vi "Teleop.vi"(10 "Match Info":T1={"Autonomous Elapsed Seconds"=0.0, "TeleOp Elapsed Seconds"=0.0, "Disabled Elapsed Seconds"=0.0, "Visited Autonomous"=FALSE, "Visited TeleOp"=FALSE, "Visited Disabled"=FALSE, "Autonomous Settings"={"Autonomous Style"=enum."Independent", "VI Refnum"=refnum}}, 11 "Call Context":T2) -> ()   [LabVIEW 2017]
doc: "This VI is called for each TeleOp packet received from the DS where the robot is not disabled. It is often used to read from the joysticks and update I/O or to update setpoints for timed control loops. It should complete and return within 20 milliseconds or it may miss DS packets."
uses:
  <vilib>/Rock Robotics/WPI/DriverStation/WPI_DriverStationDerivedRobotMode.ctl
  <vilib>/Rock Robotics/WPI/DriverStation/WPI_DriverStationMatch Info.ctl
  Public/Documents/Cross The Road Electronics/Phoenix-LabVIEW/Pigeon IMU/CTRE_PigeonIMU_PigeonState.ctl
  <vilib>/Rock Robotics/WPI/Utilities/WPI_GetSetVariantRefNum.vi
  Public/Documents/Cross The Road Electronics/Phoenix-LabVIEW/Pigeon IMU/CTRE_PigeonIMU_GetFusedHeading.vi
  Public/Documents/Cross The Road Electronics/Phoenix-LabVIEW/Pigeon IMU/CTRE_PigeonIMU_GetTempStateUpTime.vi
  Public/Documents/Cross The Road Electronics/Phoenix-LabVIEW/Pigeon IMU/CTRE_PigeonIMU_GetRawGyro.vi
  <vilib>/Rock Robotics/Network Tables/NT Write Numeric Array.vi
panel:
  in  "D Gain":dbl=0.0004 format="%#_13g"
  in  "P Gain":dbl=0.04 format="%#_13g"
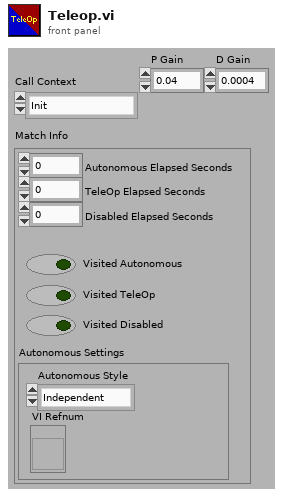
[diagram p1: front panel]
types:
  T1 = typedef "WPI_DriverStationMatch Info.ctl" = cluster{"Autonomous Elapsed Seconds":dbl, "TeleOp Elapsed Seconds":dbl, "Disabled Elapsed Seconds":dbl, "Visited Autonomous":bool, "Visited TeleOp":bool, "Visited Disabled":bool, "Autonomous Settings":cluster{"Autonomous Style":enum16{"Iterative", "Independent"}, "VI Refnum":refnum<vi>}}
  T2 = typedef "WPI_DriverStationDerivedRobotMode.ctl" = enum16{"Init", "Execute", "Stop"}
  T3 = typedef "WPI_RobotDriveDevRef.ctl" = cluster{"DevStatus":errorcluster, "Motors[]":T4[], "Square Inputs":bool, "Max Output":dbl}
  T4 = typedef "WPI_MotorControlDeviceRef.ctl" = cluster{"DeviceStatus":errorcluster, "Type":T5, "PWM":cluster{"PWM Channel":T6, "DeadBand":T7}, "CAN":cluster{"Device Number":u8, "SetOutput VI Ref":variant, "GetOutput VI Ref":variant, "Enable VI Ref":variant, "Disable VI Ref":variant, "Data":variant}, "Invert":bool, "DIO PWM":cluster{"PWM \"Enable\" Channel":T6, "DIOChannel":T8, "PWM Rate":dbl}}
  T5 = typedef "WPI_MotorControlType.ctl" = enum16{"PWM", "CAN", "DIO PWM"}
  T6 = typedef "FPGA_DIOPWMChannel.ctl" = enum8{"PWM 0", "PWM 1", "PWM 2", "PWM 3", "PWM 4", "PWM 5", "PWM 6", "PWM 7", "PWM 8", "PWM 9", "PWM MXP 0", "PWM MXP 1", "PWM MXP 2", "PWM MXP 3", "PWM MXP 4", "PWM MXP 5", "PWM MXP 6", "PWM MXP 7", "PWM MXP 8", "PWM MXP 9", "Invalid"}
  T7 = typedef "WPI_PWMDeadband.ctl" = cluster{"Name":string, "maxPositivePwm":i32, "minPositivePwm":i32, "centerPwm":i32, "maxNegativePwm":i32, "minNegativePwm":i32, "angularRange":u16}
  T8 = typedef "FPGA_DIOChannel.ctl" = enum8{"DIO 0", "DIO 1", "DIO 2", "DIO 3", "DIO 4", "DIO 5", "DIO 6", "DIO 7", "DIO 8", "DIO 9", "DIO MXP 0", "DIO MXP 1", "DIO MXP 2", "DIO MXP 3", "DIO MXP 4", "DIO MXP 5", "DIO MXP 6", "DIO MXP 7", "DIO MXP 8", "DIO MXP 9", "DIO MXP 10", "DIO MXP 11", "DIO MXP 12", "DIO MXP 13", "DIO MXP 14", "DIO MXP 15", "SPI Port CS1", "SPI Port CS2", "SPI Port CS3", "SPI Port MISO", "SPI Port MOSI", "Invalid"}
  T9 = typedef "WPI_JoystickDevRef.ctl" = cluster{"Device":T10}
  T10 = typedef "WPI_JoystickDeviceEnum.ctl" = enum16{"USB 0", "USB 1", "USB 2", "USB 3", "USB 4", "USB 5"}
  T11 = typedef "CTRE_PigeonIMU_DeviceRef.ctl" = cluster{"DeviceStatus":errorcluster, "Device Number":u8, "Type":T12, "Device ID":u32, "Handle":u64, "UsageFrame":u32, "Library Path":path}
  T12 = typedef "CTRE_PigeonIMU_ConnectionType.ctl" = u32
  T13 = typedef "CTRE_PigeonIMU_PigeonState.ctl" = enum16{"NoComm", "Initializing", "Ready", "UserCalibration"}
  T14 = cluster{"Heading":dbl, "Valid?":bool, "Fusing?":bool}
  T15 = typedef "CTRE_PigeonIMU_CalibrationMode.ctl" = u16
  T16 = cluster{"CurrentMode":T15, "LastCalError":i32, "CalBooting?":bool, "PigeonState":T13, "UpTime":u32, "Temp. (C)":dbl, "Temp Compensation Event Count":u32, "No Motion Event Count":u32}
  T17 = cluster{"X":dbl, "Y":dbl, "Z":dbl, "Magnitude":dbl}
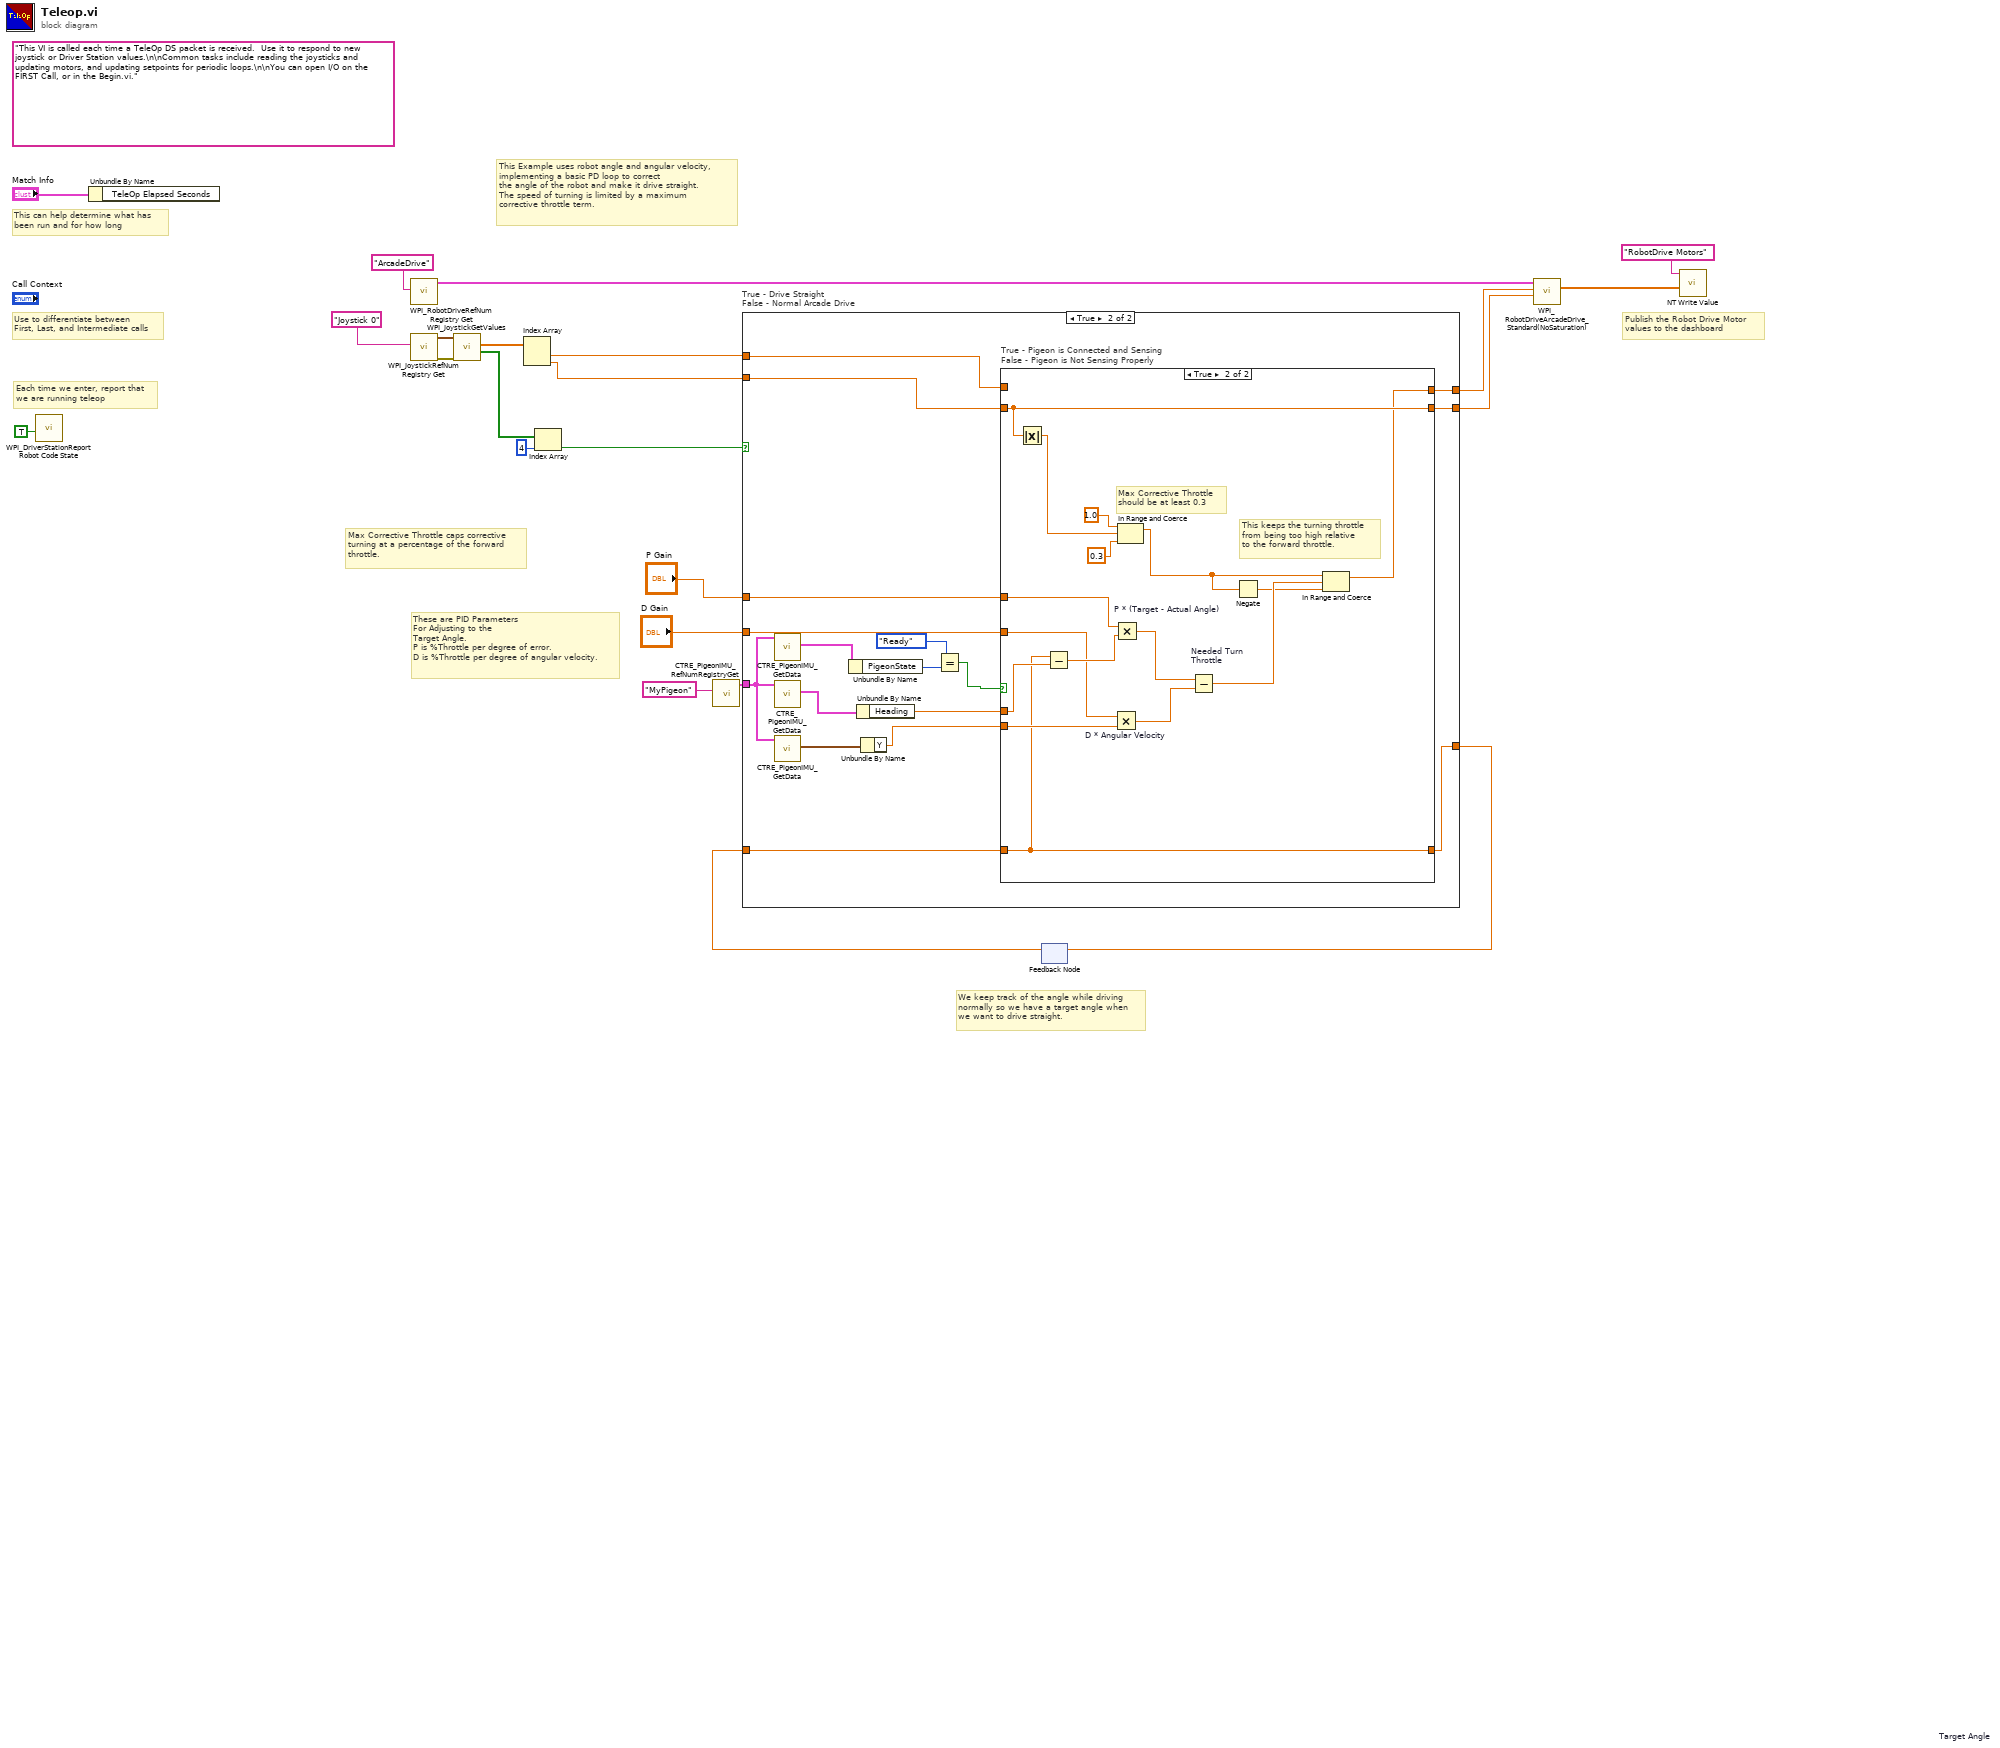
[diagram p0: block diagram]
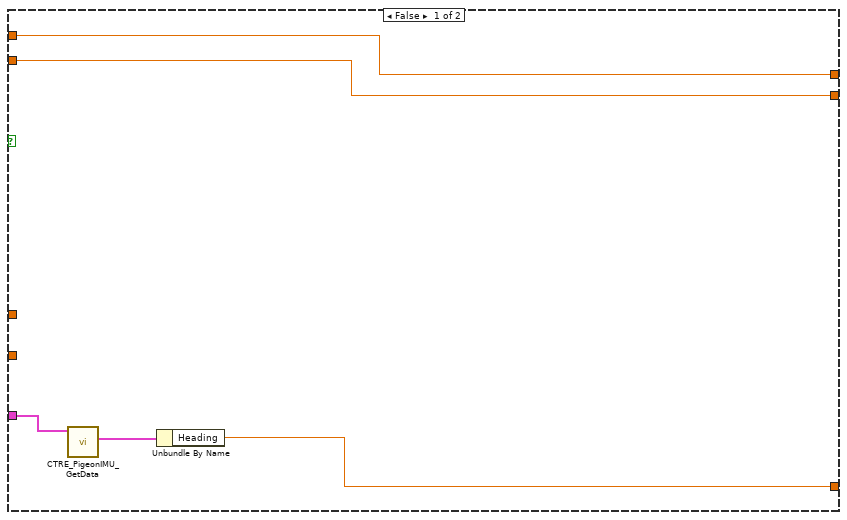
[diagram p2: hidden frame]
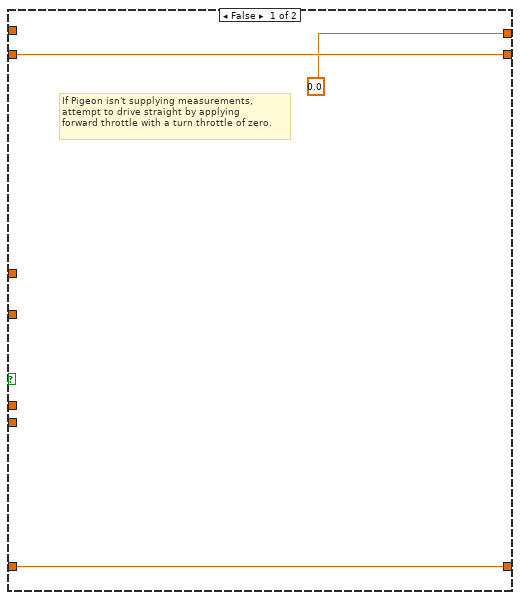
[diagram p3: hidden frame]
diagram:
  (unwired) "This VI is called each time a TeleOp DS packet is received.  Use it to respond to new joystick or Driver Station values.\n\nCommon tasks include reading the joysticks and updating motors, and updating setpoints for periodic loops.\n\nYou can open I/O on the FIRST Call, or in the Begin.vi."
  # "This Example uses robot angle and angular velocity, \nimplementing a basic PD loop to correct\nthe angle of the robot and make it drive straight.\nThe speed of turning is limited by a maximum \ncorrective throttle term."
  # "Max Corrective Throttle caps corrective\nturning at a percentage of the forward\nthrottle."
  # "We keep track of the angle while driving\nnormally so we have a target angle when\nwe want to drive straight."
  # "These are PID Parameters\nFor Adjusting to the\nTarget Angle.\nP is %Throttle per degree of error.\nD is %Throttle per degree of angular velocity."
  # "Publish the Robot Drive Motor\nvalues to the dashboard"
  # "Each time we enter, report that\nwe are running teleop"
  # "Use to differentiate between\nFirst, Last, and Intermediate calls"
  # "This can help determine what has\nbeen run and for how long"
  n1 = call <vilib>:"WPI_DriverStationReport Robot Code State.vi"("TeleOp"=TRUE ("Autonomous")) -> ()  [unwired: 10 in, 1 out]
  n2 = Unbundle By Name("Match Info") -> ()  [unwired: 1 out]
  n3 = call <vilib>:"WPI_RobotDriveRefNum Registry Get.vi"("refnum name"="ArcadeDrive") -> ("RobotDriveDevRef"=w21:T3)  [unwired: 1 in, 9 out]
  n4 = call <vilib>:"WPI_JoystickRefNum Registry Get.vi"("refnum name"="Joystick 0") -> ("error out"=w7:errorcluster, "JoystickDevRef"=w19:T9)  [unwired: 1 in, 8 out]
  n5 = call <vilib>:"WPI_JoystickGetValues.vi"("error in (no error)"=w7, "JoystickDevRef"=w19) -> ("Buttons"=w10:bool[], "Axes"=w17:dbl[])  [unwired: 5 in, 3 out]
  n6 = Index Array(array=w17) -> (element #1=w14:dbl, element #2=w13:dbl)  [unwired: 2 in]
  n7 = Index Array(array=w10, index=4) -> (element=w8:bool)
  n8 = call "CTRE_PigeonIMU_RefNumRegistryGet.vi"("refnum name"="MyPigeon") -> ("PigeonIMUDevRef"=w2:T11)  [unwired: 9 in, 1 out]
  n9 = feedback #1 "Target Angle"() -> (w3:dbl)  [unwired: 1 in]
  n10 = case "True - Drive Straight\nFalse - Normal Arcade Drive" shown="True" w8 {
    tunnel: w14 -> [w28 w45]
    tunnel: w13 -> [w27 w44]
    tunnel: [w28 w42] -> w11
    tunnel: [w27 w43] -> w12
    tunnel: w2 -> [w25 w29]
    tunnel: "P Gain" -> [_ w39]
    tunnel: "D Gain" -> [_ w38]
    tunnel: [w26 w37] -> w4
    tunnel: w3 -> [_ w40]
    frame False {
      n11 = call-poly "CTRE_PigeonIMU_GetData.vi"("PigeonIMUDevRef"=w25) -> ("Fused Heading"=w24:T14)  [unwired: 8 in, 2 out]
      n12 = Unbundle By Name(w24) -> ("Heading"=w26:dbl)
    }
    frame True {
      n13 = call-poly "CTRE_PigeonIMU_GetData.vi"("PigeonIMUDevRef"=w29) -> ("Temp/State/UpTime"=w33:T16)  [unwired: 8 in, 2 out]
      n14 = call-poly "CTRE_PigeonIMU_GetData.vi"("PigeonIMUDevRef"=w29) -> ("Fused Heading"=w36:T14)  [unwired: 8 in, 2 out]
      n15 = call-poly "CTRE_PigeonIMU_GetData.vi"("PigeonIMUDevRef"=w29) -> ("Gyro DPS"=w35:T17)  [unwired: 8 in, 2 out]
      n16 = Unbundle By Name(w33) -> ("PigeonState"=w32:T13)
      n17 = Unbundle By Name(w36) -> ("Heading"=w41:dbl)
      n18 = Unbundle By Name(w35) -> ("Y"=w34:dbl)
      n19 = Equal?(x=CTRE_PigeonIMU_PigeonState."Ready", y=w32) -> (x = y?=w31:bool)
      n20 = case "True - Pigeon is Connected and Sensing\nFalse - Pigeon is Not Sensing Properly" shown="True" w31 {
        tunnel: w45 -> [_ _]
        tunnel: w44 -> [w48 w57]
        tunnel: [w48 w57] -> w43
        tunnel: [0.0 ("upper limit") w51] -> w42
        tunnel: w41 -> [_ w64]
        tunnel: w40 -> [w46 w50]
        tunnel: w34 -> [_ w61]
        tunnel: w39 -> [_ w62]
        tunnel: w38 -> [_ w60]
        tunnel: [w46 w50] -> w37
        frame False {
          # "If Pigeon isn't supplying measurements,\nattempt to drive straight by applying\nforward throttle with a turn throttle of zero."
        }
        frame True {
          # "This keeps the turning throttle\nfrom being too high relative\nto the forward throttle."
          # "Max Corrective Throttle\nshould be at least 0.3"
          n21 = Absolute Value(x=w57) -> (abs(x)=w49:dbl)
          n22 = Subtract(x=w50, y=w64) -> (x-y=w63:dbl)
          n23 = Multiply "D * Angular Velocity"(x=w60, y=w61) -> (x*y=w58:dbl)
          n24 = Multiply "P * (Target - Actual Angle)"(x=w62, y=w63) -> (x*y=w59:dbl)
          n25 = In Range and Coerce(upper limit=1.0, x=w49, lower limit=0.3) -> (coerced(x)=w53:dbl)  [unwired: 1 out]
          n26 = Subtract "Needed Turn \nThrottle"(x=w59, y=w58) -> (x-y=w54:dbl)
          n27 = Negate(x=w53) -> (-x=w52:dbl)
          n28 = In Range and Coerce(upper limit=w53, x=w54, lower limit=w52) -> (coerced(x)=w51:dbl)  [unwired: 1 out]
        }
      }
    }
  }
  n29 = feedback-in #1(w4) -> ()
  n30 = call <vilib>:"WPI_RobotDriveArcadeDrive_Standard(NoSaturation).vi"("Y axis value"=w12, "X axis value"=w11, "RobotDriveDevRef"=w21) -> ("Motor Values"=w16:dbl[])  [unwired: 1 in, 7 out]
  n31 = call-poly <vilib>:"NT Write Value.vi"("Numeric Array"=w16, "Name"="RobotDrive Motors") -> ()  [unwired: 9 in, 1 out]
